vi "Convert CAN Frame (Extended Data) to U32.vi"(7 "CAN FRAME TIMED":T1 {"payload" format="%x"; "timestamp" format="%<%.7X\n%x>T"; "type" items=["CAN Data"=0, "CAN Remote"=1, "CAN Bus Error"=2, "CAN 2.0 Data"=8, "CAN FD Data"=16, "CAN FD+BRS Data"=24, "J1939 Data"=192, "Delay"=224, "Log Trigger"=225, "Start Trigger"=226]; "identifier" format="%x"}) -> (8 "Data":u32[](array[numeric]))   [LabVIEW 2019, in "J1939 Utilities.lvlib"]
uses:
  J1939 Utilities.lvlib
  <vilib>/xnet/xnet.llb/XNET Frame CAN.ctl
  <vilib>/xnet/xnet.llb/XNET Frame Type CAN.ctl
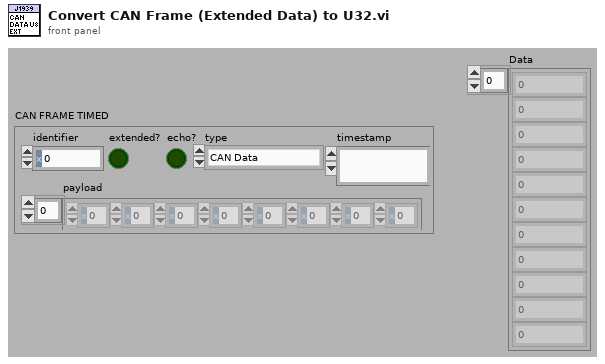
[diagram p1: front panel]
types:
  T1 = typedef "XNET Frame CAN.ctl" = cluster{"timestamp":timestamp, "payload":u8[], "identifier":u32, "type":T2, "extended?":bool, "echo?":bool}
  T2 = typedef "XNET Frame Type CAN.ctl" = u8
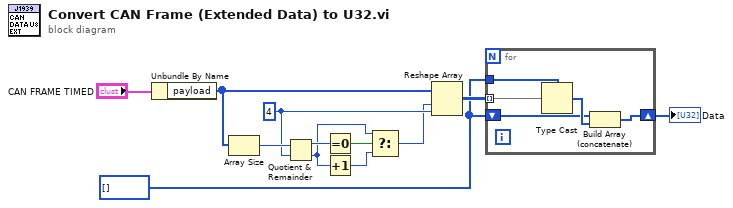
[diagram p0: block diagram]
diagram:
  w2 = u32[] [] ("Data")
  w10 = 4 ("dimension size")
  n1 = Unbundle By Name("CAN FRAME TIMED") -> ("payload"=w12:u8[])
  n2 = Array Size(array=w12) -> (size(s)=w11:i32)
  n3 = Quotient & Remainder(x=w11, y=w10) -> (x-y*floor(x/y)=w9:i32, floor(x/y)=w7:i32)
  n4 = Equal To 0?(x=w9) -> (x = 0?=w8:bool)
  n5 = Increment(x=w7) -> (x+1=w6:i32)
  n6 = Select(t=w7, s=w8, f=w6) -> (s? t:f=w5:i32)
  n7 = Reshape Array(w12, w5, w10) -> (w4:u8[][])
  n8 = for {
    tunnel: w4 -> [w17] mode=indexing
    shift-right: [w15] -> w3
    shift-left: w2 -> [w14]
    tunnel: w2 -> [w13]
    n9 = Type Cast(type=w13, x=w17) -> (*(type *) &x=w16:u32[])
    n10 = Build Array (concatenate)(w14, w16) -> (w15:u32[])
  }
  "Data" <- w3
